vi "zad_dom.vi"() -> ()   [LabVIEW 2017]
panel:
  in  "stop":bool
  out "Boolean 12":bool
  out "Boolean 11":bool
  out "Boolean 10":bool
  out "Boolean 9":bool
  out "Boolean 8":bool
  out "Boolean 7":bool
  in  "switch when pressed":bool
  in  "latch until released":bool
  in  "latch when released":bool
  in  "latch when pressed":bool
  in  "switch until released":bool
  in  "switch when released":bool
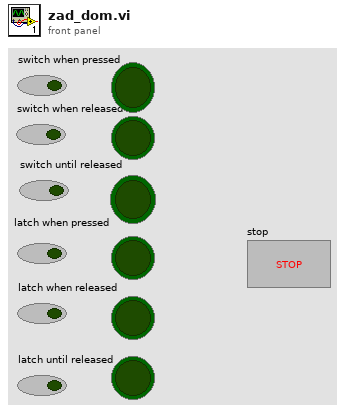
[diagram p1: front panel]
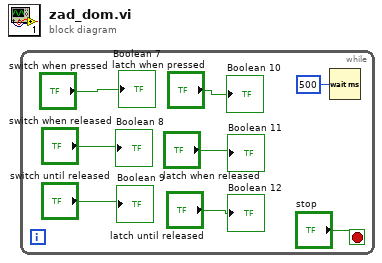
[diagram p0: block diagram]
diagram:
  n1 = while {
    stop <- "stop" stop-if-true
    n2 = Wait (ms)(milliseconds to wait=u32 500) -> ()  [unwired: 1 out]
    "Boolean 7" <- "switch when pressed"
    "Boolean 9" <- "switch until released"
    "Boolean 10" <- "latch when pressed"
    "Boolean 8" <- "switch when released"
    "Boolean 11" <- "latch when released"
    "Boolean 12" <- "latch until released"
  }
